vi "Display and Log Custom Device Error.vi"(8 "error out":errorcluster, 9 "Note (empty)":string, 10 "Your code's public name":string, 11 "Custom Device? (T)":bool=TRUE) -> ()   [LabVIEW 2015, in "VS Inline Async API.lvlib" / "VS Inline Async API.lvclass"]
uses:
  VS Inline Async API.lvclass
  <vilib>/NI Veristand/Custom Device Tools/Custom Device Utility Library/Custom Device Utility Library.lvlib
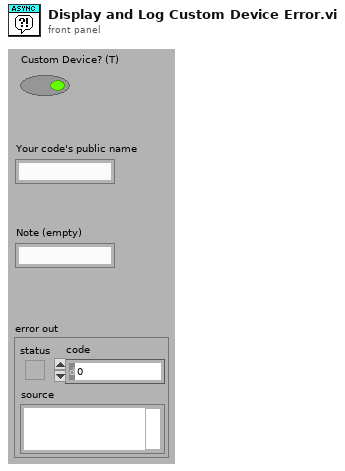
[diagram p1: front panel]
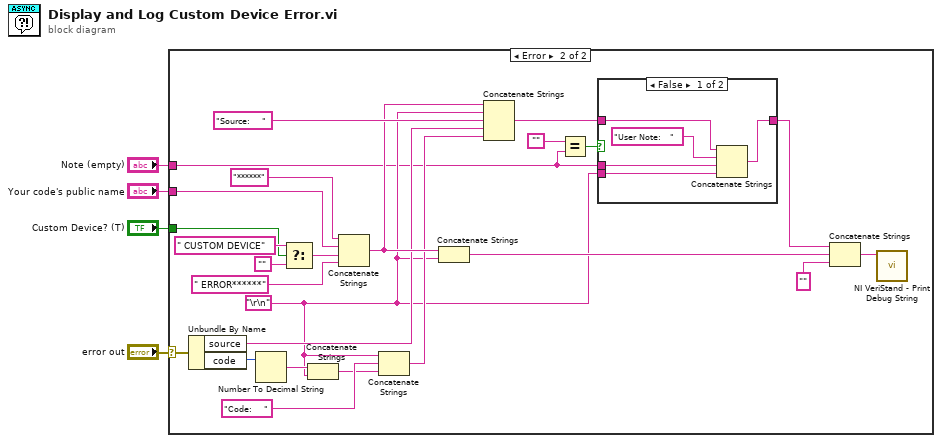
[diagram p0: block diagram]
diagram:
  n1 = case shown="Error" "error out" {
    selector: "error out" -> [_ w29]
    tunnel: "Custom Device? (T)" -> [_ w17]
    tunnel: "Your code's public name" -> [_ w8]
    tunnel: "Note (empty)" -> [_ w6]
    frame No Error {
    }
    frame Error {
      w7 = "\r\n"
      n2 = Unbundle By Name(w29) -> ("source"=w16:string, "code"=w10:i32)
      n3 = Number To Decimal String(number=w10) -> (decimal integer string=w26:string)  [unwired: 1 in]
      n4 = Select(t=" CUSTOM DEVICE" ("String"), s=w17, f="") -> (s? t:f=w18:string)
      n5 = Concatenate Strings(w26, w7) -> (w9:string)
      n6 = Concatenate Strings("******" ("String"), w8, w18, " ERROR******" ("String")) -> (w21:string)
      n7 = Concatenate Strings(w7, "Code:    " ("String"), w9) -> (w15:string)
      n8 = Concatenate Strings(w21, w7) -> (w12:string)
      n9 = Concatenate Strings(w21, w7, "Source:    " ("String"), w16, w15) -> (w14:string)
      n10 = Equal?(x="", y=w6) -> (x = y?=w19:bool)
      n11 = case shown="False" w19 {
        tunnel: w6 -> [w33 _]
        tunnel: w7 -> [w32 _]
        tunnel: w14 -> [w31 w35]
        tunnel: [w30 w35] -> w13
        frame False {
          n12 = Concatenate Strings(w31, "User Note:   " ("string"), w33, w32) -> (w30:string)
        }
        frame True {
        }
      }
      n13 = Concatenate Strings(w13, w12, "" ("Message")) -> (w5:string)
      n14 = call <vilib>:"NI VeriStand - Print Debug String.vi"("Message"=w5) -> ()  [unwired: 10 in, 1 out]
    }
  }
